vi "Plot calc y axis visibility.vi"(8 "error in (no error)":errorcluster, 10 "top array":T1[](array[typedef]), 11 "Plot":refnum<vi>) -> (0 "error out":errorcluster, 1 "Right axis visible?":bool, 2 "Left axis visible?":bool, 3 "Plot":refnum<vi>, 4 "Multi-Y?":bool)   [LabVIEW 2021, in "RocketPlot.lvlib"]
uses:
  RocketPlot.lvlib
  TypeDefs/Plot top row.ctl
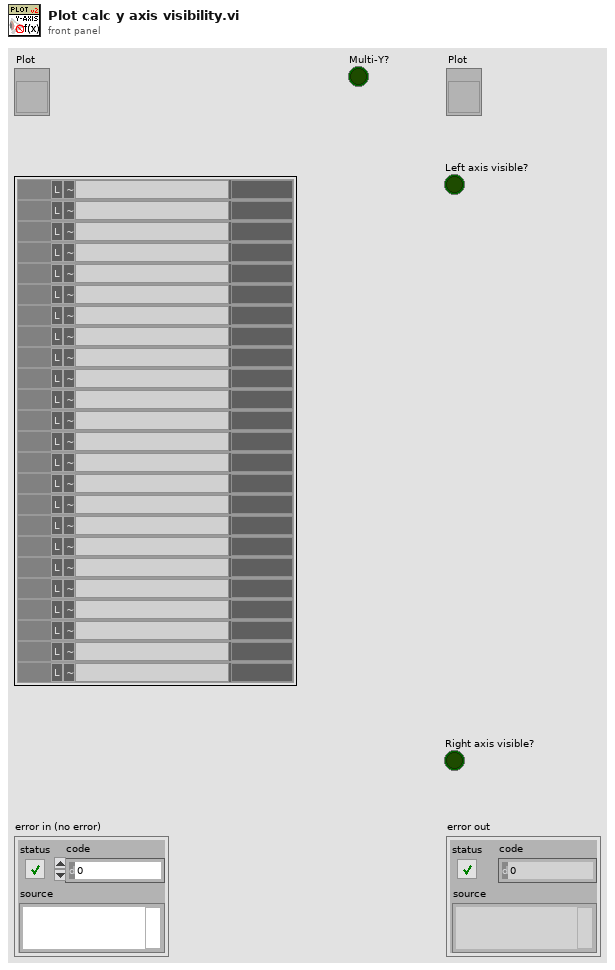
[diagram p1: front panel]
types:
  T1 = typedef "RocketPlot.lvlib/Plot top row.ctl" = cluster{"PID":string, "index":i32, "PID color":u32, "right axis?":bool, "Flatline?":bool, "Numeric color":u32, "Data":string, "Flat":string}
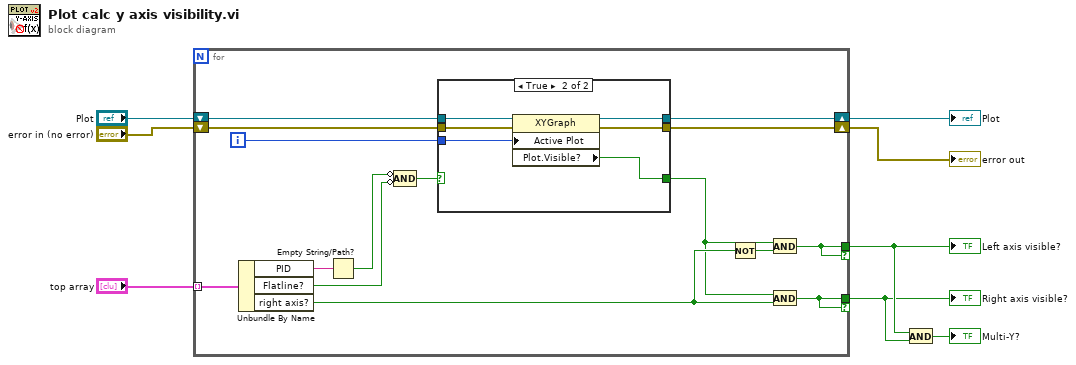
[diagram p0: block diagram]
diagram:
  n1 = for {
    tunnel: "top array" -> [w23] mode=indexing
    tunnel: [w18] -> w3 if=w18
    tunnel: [w19] -> w2 if=w19
    shift-right: [w11] -> w4
    shift-left: "Plot" -> [w15]
    shift-right: [w10] -> w5
    shift-left: "error in (no error)" -> [w9]
    i -> [w14]
    n2 = Unbundle By Name(w23) -> ("PID"=w22:string, "Flatline?"=w20:bool, "right axis?"=w16:bool)
    n3 = Empty String/Path?(string/path=w22) -> (empty?=w21:bool)
    n4 = Compound Arithmetic op=AND(invert w21, invert w20) -> (w13:bool)
    n5 = case shown="True" w13 {
      selector: w13 -> [w26 _]
      tunnel: w15 -> [w25 w32]
      tunnel: w14 -> [_ w31]
      tunnel: [w26 w30] -> w12
      tunnel: [w25 w29] -> w11
      tunnel: [w24 w28] -> w10
      tunnel: w9 -> [w24 w27]
      frame False {
      }
      frame True {
        n6 = property class="XYGraph"(reference=w32, error in=w27, "Active Plot"=w31) -> (reference out=w29:refnum<vi>, error out=w28:errorcluster, "Plot.Visible?"=w30:bool)
      }
    }
    n7 = Not(x=w16) -> (.not. x?=w17:bool)
    n8 = And(x=w12, y=w17) -> (x .and. y?=w18:bool)
    n9 = And(x=w12, y=w16) -> (x .and. y?=w19:bool)
  }
  "error out" <- w5
  "Plot" <- w4
  "Left axis visible?" <- w3
  "Right axis visible?" <- w2
  n10 = And(x=w3, y=w2) -> (x .and. y?=→"Multi-Y?":bool)
